vi "ApplyVIPC.vi"   [LabVIEW 2020]
uses:
  <vilib>/Wiresmith Technology/G CLI/CLI Class/CLI.lvclass
  <vilib>/JKI/VIPM API/VIPM API_vipm_api.lvlib
types:
  T1 = enum32{"Invalid", "Standard", "Closed", "Hidden", "Minimized", "Maximized"}
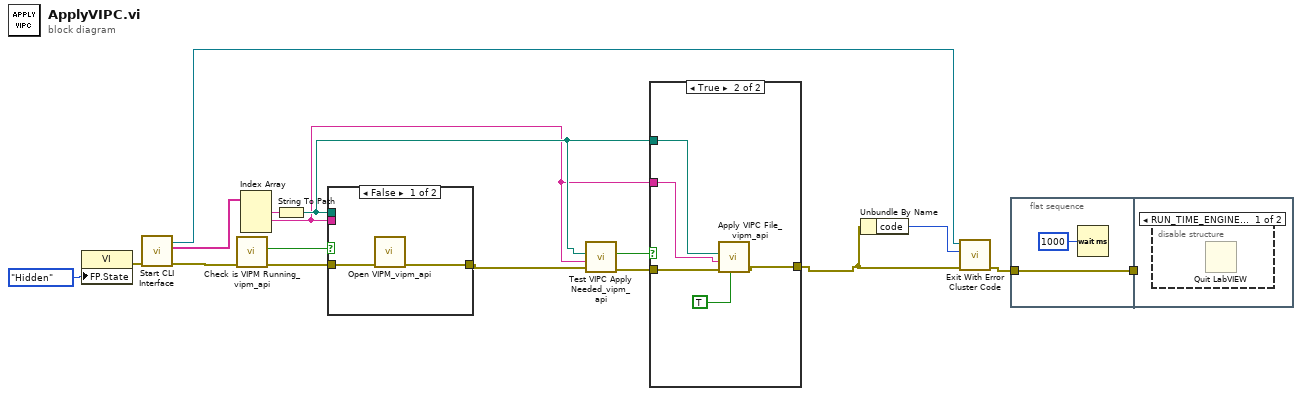
[diagram p0: block diagram]
diagram:
  n1 = property class="VI"("FP.State"=T1."Hidden" ("Front Panel Window:State")) -> (error out=w16:errorcluster)  [unwired: 2 in, 1 out]
  n2 = call <vilib>:"Start CLI Interface.vi"("error in (no error)"=w16) -> ("error out"=w8:errorcluster, "Custom Parameters"=w12:string[], "CLI out"=w15:refnum<class "CLI.lvclass">)  [unwired: 7 in, 1 out]
  n3 = call <vilib>:"Check is VIPM Running_vipm_api.vi"("error in (no error)"=w8) -> ("error out"=w14:errorcluster, "is Running"=w13:bool)  [unwired: 9 in]
  n4 = Index Array(array=w12) -> (element #1=w7:string, element #2=w3:string)  [unwired: 3 in, 1 out]
  n5 = String To Path(string=w7) -> (path=w4:path)
  n6 = case shown="False" w13 {
    tunnel: w14 -> [w19 w20]
    tunnel: w4 -> [_ _]
    tunnel: w3 -> [_ _]
    tunnel: [w18 w20] -> w2
    frame False {
      n7 = call <vilib>:"Open VIPM_vipm_api.vi"("error in (no error)"=w19) -> ("error out"=w18:errorcluster)  [unwired: 10 in]
    }
    frame True {
    }
  }
  n8 = call <vilib>:"Test VIPC Apply Needed_vipm_api.vi"("error in (no error)"=w2, "LabVIEW Version (use vipc version)"=w3, "VIPC File Path"=w4) -> ("error out"=w5:errorcluster, "Need to Apply?"=w6:bool)  [unwired: 6 in, 1 out]
  n9 = case shown="True" w6 {
    tunnel: w5 -> [w21 w25]
    tunnel: [w21 w24] -> w1
    tunnel: w4 -> [_ w23]
    tunnel: w3 -> [_ w22]
    frame False {
    }
    frame True {
      n10 = call <vilib>:"Apply VIPC File_vipm_api.vi"("quiet? (T)"=TRUE, "error in (no error)"=w25, "LabVIEW Version"=w22, "VIPC File"=w23) -> ("error out"=w24:errorcluster)  [unwired: 7 in]
    }
  }
  n11 = Unbundle By Name(w1) -> ("code"=w9:i32)
  n12 = call <vilib>:"Exit With Error Cluster Code.vi"("error in (no error)"=w1, "No Error Code (0)"=w9, "CLI in"=w15) -> ("error out"=w10:errorcluster)  [unwired: 8 in]
  n13 = flat-sequence {
    tunnel: w10 -> [w28]
    tunnel: [w28] -> w11
    tunnel: w11 -> [_]
    frame #0 {
      n14 = Wait (ms)(milliseconds to wait=u32 1000) -> ()  [unwired: 1 out]
    }
    frame #1 {
      n15 = disable-structure shown="RUN_TIME_ENGINE==True" {
        frame condition #0 {
          n16 = Quit LabVIEW() -> ()  [unwired: 1 in]
        }
        frame condition #1 (active) {
        }
      }
    }
  }
